vi "draw.vi"(0 "reference":refnum<class "NoteEdge.lvclass">, 1 "graphics":refnum<class "Graphics.lvclass">, 5 "error in (no error)":errorcluster) -> (14 "reference out":refnum<class "NoteEdge.lvclass">, 19 "error out":errorcluster)   [LabVIEW 2016, in "NoteEdge.lvclass"]
doc: "public void draw(Graphics2D g2, Point2D p, Point2D q)"
uses:
  <resource>/Framework/Providers/Open_GDS/UML/NoteEdge_class/NoteEdge.lvclass
  <resource>/Framework/Providers/Open_GDS/UML/Graphics_class/Graphics.lvclass
  <resource>/Framework/Providers/Open_GDS/UML/Graphics_class/StrokeType.ctl
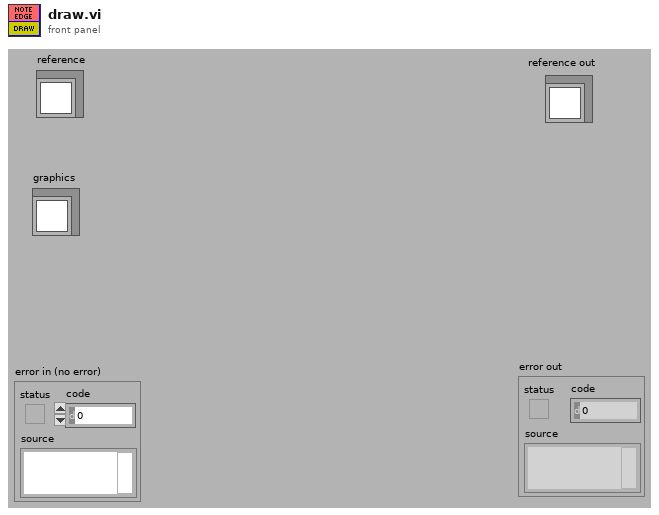
[diagram p1: front panel]
types:
  T1 = typedef "Graphics.lvclass/StrokeType.ctl" = enum16{"USE_DEFAULT", "SOLID", "DOTTED"}
  T2 = typedef "Point Point2D.ctl" = cluster{"x":dbl, "y":dbl}
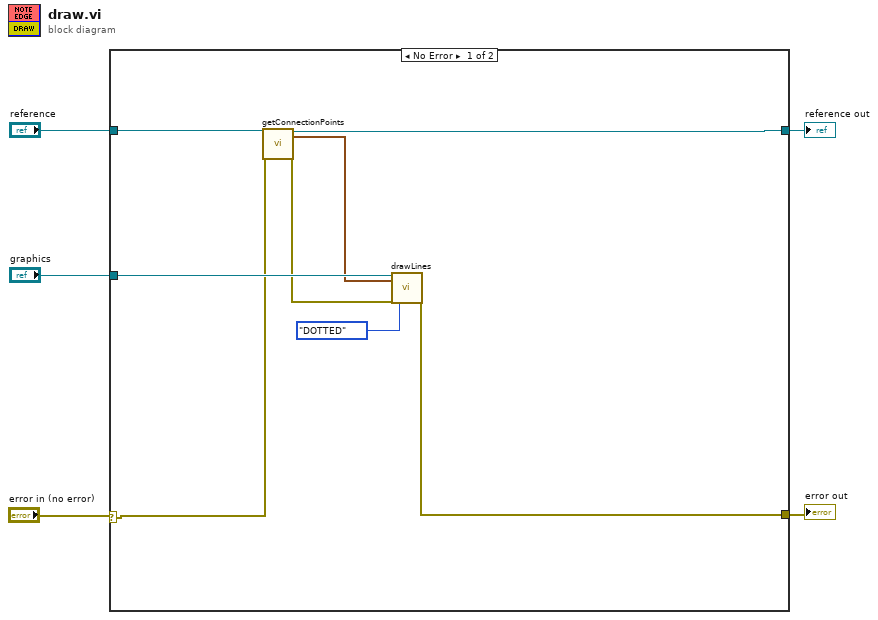
[diagram p0: block diagram]
diagram:
  n1 = case shown="No Error" "error in (no error)" {
    selector: "error in (no error)" -> [w6 w14]
    tunnel: "reference" -> [w13 w15]
    tunnel: [w12 w14] -> w4
    tunnel: [w11 w15] -> w3
    tunnel: "graphics" -> [w10 _]
    frame No Error {
      n2 = call-dynamic "getConnectionPoints.vi"("reference"=w13, "error in (no error)"=w6) -> ("reference out"=w11:refnum<class "NoteEdge.lvclass">, "connectionPoints"=w9:T2[], "error out"=w8:errorcluster)  [unwired: 15 in]
      n3 = call <resource>:"drawLines.vi"("reference"=w10, "points"=w9, "error in (no error)"=w8, "stroke"=StrokeType."DOTTED") -> ("error out"=w12:errorcluster)  [unwired: 3 in, 12 out]
    }
    frame Error {
    }
  }
  "reference out" <- w3
  "error out" <- w4
